vi "Actor Core.vi"(8 "error in":errorcluster, 11 "LF2R IDE in":refnum<class "LF2R IDE.lvclass">) -> (0 "error out":errorcluster, 3 "Actor out":refnum<class "Actor.lvclass">)   [LabVIEW 2018, in "LF2R IDE.lvlib" / "LF2R IDE.lvclass"]
doc: "The user interface for this panel.\n\n----\nPlease see the following web address for additional documentation and tutorial information:\nhttp://www.mooregoodideas.com/mgi-panel-manager/\n\nAuthor: Derek Trepanier\n\nCopyright (c) 2018, Moore Good Ideas, Inc.\n\nAll rights reserved.\n\nRedistribution and use in source and binary forms, with or without modification, are permitted provided that the following conditions are met:\n\n * Redistributions of source code must retain the above copyright notice, this list of conditions and the following disclaimer.\n * Redistributions in binary form must reproduce the above copyright notice, this list of conditions and the following disclaimer in the documentation and/or other materials provided with the distribution.\n * Neither the name of Moore Good Ideas, Inc. nor the names of its contributors may be used to endorse or promote products derived from this software without specific prior written permission.\n\nTHIS SOFTWARE IS PROVIDED BY THE COPYRIGHT HOLDERS AND CONTRIBUTORS \"AS IS\" AND ANY EXPRESS OR IMPLIED WARRANTIES, INCLUDING, BUT NOT LIMITED TO, THE IMPLIED WARRANTIES OF MERCHANTABILITY AND FITNESS FOR A PARTICULAR PURPOSE ARE DISCLAIMED. IN NO EVENT SHALL THE COPYRIGHT OWNER OR CONTRIBUTORS BE LIABLE FOR ANY DIRECT, INDIRECT, INCIDENTAL, SPECIAL, EXEMPLARY, OR CONSEQUENTIAL DAMAGES (INCLUDING, BUT NOT LIMITED TO, PROCUREMENT OF SUBSTITUTE GOODS OR SERVICES; LOSS OF USE, DATA, OR PROFITS; OR BUSINESS INTERRUPTION) HOWEVER CAUSED AND ON ANY THEORY OF LIABILITY, WHETHER IN CONTRACT, STRICT LIABILITY, OR TORT (INCLUDING NEGLIGENCE OR OTHERWISE) ARISING IN ANY WAY OUT OF THE USE OF THIS SOFTWARE, EVEN IF ADVISED OF THE POSSIBILITY OF SUCH DAMAGE."
uses:
  LF2R IDE.lvclass
  C:/Program Files (x86)/National Instruments/LabVIEW 2018/vi.lib/MGI/Panel Manager/Panel Actor/Panel Actor/Panel Actor.lvclass
  <vilib>/ActorFramework/Actor/Actor.lvclass
  LF2R IDE.lvclass/LF2R IDE.ctl
  <vilib>/MGI/Panel Manager/Panel Actor/Panel Actor/Panel Actor.lvclass
  D:/project/hobby/LabVIEW/LF2R/LabVIEW/Source/ScintillaNET/dll/ScintillaNET.dll
  ScintillaNET/dll/ScintillaNET.dll
panel:
  in  "File Path":path
  in  "Script":refnum<k24>(container)
  in  "Numeric":u32
  in  "Load Pic":bool
  in  "Go To":u16(ring)
  in  "Tab Control":T1(tab)
  in  "sound":string
  in  "basic_dvz":i32 caption="dvz"
  in  "basic_dvy":i32 caption="dvy"
  in  "basic_dvx":i32 caption="dvx"
  in  "basic_centery":i32 caption="centery"
  in  "basic_centerx":i32 caption="centerx"
  in  "basic_next":u32 caption="next"
  in  "basic_wait":u32 caption="wait"
  in  "basic_state":u32 caption="state"
  in  "basic_pic":u32 caption="pic"
  in  "To Next Frame":bool
  in  "basic_hit_Da":u32 caption="hit_Da"
  in  "basic_mp":i32 caption="mp"
  in  "basic_hit_Fa":u32 caption="hit_Fa"
  in  "basic_hit_Fj":u32 caption="hit_Fj"
  in  "basic_hit_Ua":u32 caption="hit_Ua"
  in  "basic_hit_Uj":u32 caption="hit_Uj"
  in  "basic_hit_Dj":u32 caption="hit_Dj"
  in  "basic_hit_ja":u32 caption="hit_ja"
  in  "basic_hit_d":u32 caption="hit_d"
  in  "basic_hit_a":u32 caption="hit_a"
  in  "basic_hit_j":u32 caption="hit_j"
  in  "bp_y":dbl caption="y"
  in  "bp_x":dbl caption="x"
  in  "w_attacking":u32 caption="attacking"
  in  "w_dvz":i32 caption="dvz"
  in  "w_dvy":i32 caption="dvy"
  in  "w_dvx":i32 caption="dvx"
  in  "w_cover":u32 caption="cover"
  in  "w_weaponact":u32 caption="weaponact"
  in  "w_y":dbl caption="y"
  in  "w_x":dbl caption="x"
  in  "w_kind":u32 caption="kind"
  in  "b_h":u32 caption="h"
  in  "b_w":u32 caption="w"
  in  "b_y":i32 caption="y"
  in  "b_x":i32 caption="x"
  in  "b_kind":u32 caption="kind"
  in  "<b> index":u32(slide) scale=0.0..10.0
  in  "i_zwidth":u32 caption="zwidth"
  in  "i_caughtact 2":u32 caption="caughtact 2"
  in  "i_catchingact 2":u32 caption="catchingact 2"
  in  "i_caughtact 1":u32 caption="caughtact 1"
  in  "i_catchingact 1":u32 caption="catchingact 1"
  in  "i_effect":u32 caption="effect"
  in  "i_injury":i32 caption="injury"
  in  "i_bdefend":i32 caption="bdefend"
  in  "i_vrest":u32 caption="vrest"
  in  "i_arest":u32 caption="arest"
  in  "i_fall":u32 caption="fall"
  in  "i_dvz":i32 caption="dvz"
  in  "i_dvy":i32 caption="dvy"
  in  "i_dvx":i32 caption="dvx"
  in  "i_h":u32 caption="h"
  in  "i_w":u32 caption="w"
  in  "i_y":i32 caption="y"
  in  "i_x":i32 caption="x"
  in  "i_kind":u32 caption="kind"
  in  "<i> index":u32(slide) scale=0.0..10.0
  in  "o_facing":i32 caption="facing"
  in  "o_oid":u32 caption="oid"
  in  "o_action":u32 caption="action"
  in  "o_kind":u32 caption="kind"
  in  "o_x":i32 caption="x"
  in  "o_y":i32 caption="y"
  in  "o_dvx":i32 caption="dvx"
  in  "o_dvy":i32 caption="dvy"
  in  "o_dvz":i32 caption="dvz"
  in  "c_cover":i32 caption="cover"
  in  "c_injury":i32 caption="injury"
  in  "c_dircontrol":i32 caption="dircontrol"
  in  "c_backhurtact":i32 caption="backhurtact"
  in  "c_fronthurtact":i32 caption="fronthurtact"
  in  "c_decrease":i32 caption="decrease"
  in  "c_hurtable":i32 caption="hurtable"
  in  "c_taction":i32 caption="taction"
  in  "c_aaction":i32 caption="aaction"
  in  "c_vaction":i32 caption="vaction"
  in  "c_y":i32 caption="y"
  in  "c_x":i32 caption="x"
  in  "c_kind":u32 caption="kind"
  in  "c_throwvx":i32 caption="throwvx"
  in  "c_throwvy":i32 caption="throwvy"
  in  "c_throwvz":i32 caption="throwvz"
  in  "c_throwinjury":i32 caption="throwinjury"
  in  "title_name":string caption="Name"
  in  "Apply Change":bool
  in  "title_num":u32 caption="Frame Num" format="%03d"
  out "Image Display":T2(plugin-control)
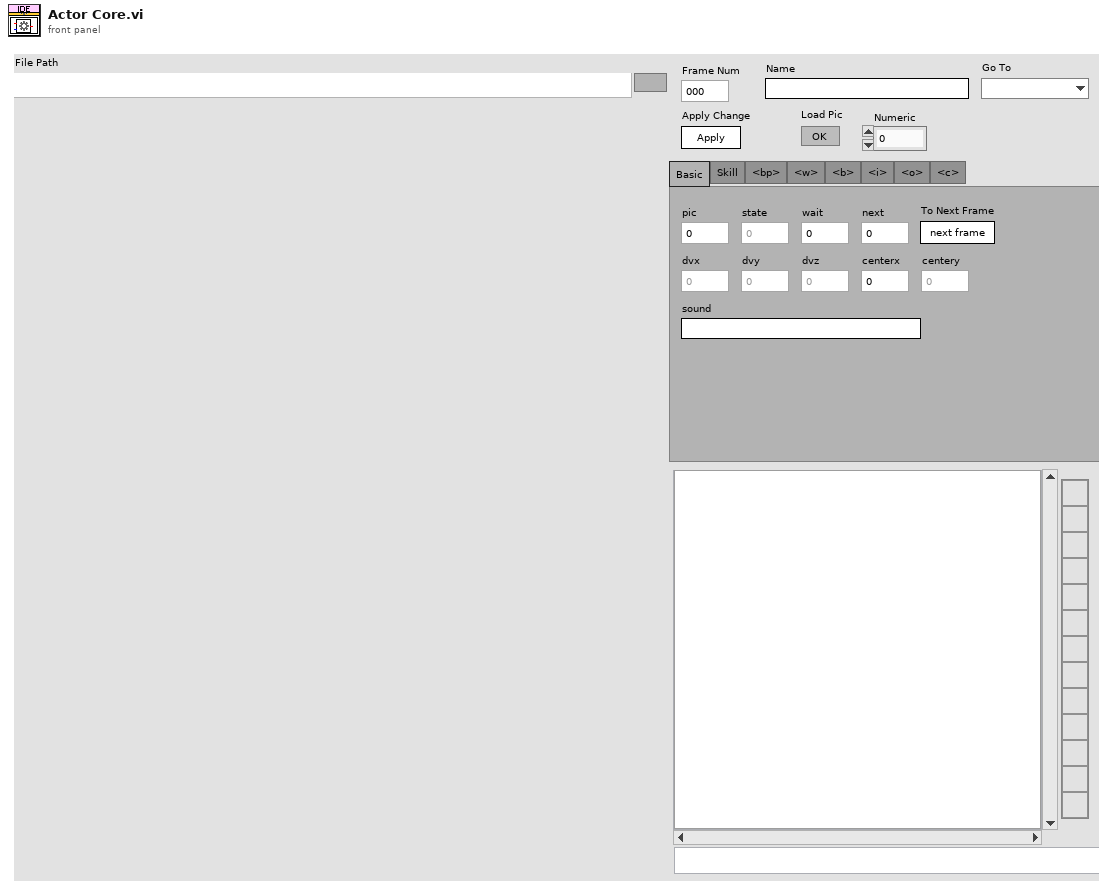
[diagram p1: front panel]
types:
  T1 = enum32{"Basic", "Skill", "<bp>", "<w>", "<b>", "<i>", "<o>", "<c>"}
  T2 = typedef "IMAQ Image.ctl" = refnum<image>
  T3 = cluster{"title_num":refnum<vi>, "title_name":refnum<vi>}
  T4 = cluster{"basic_pic":refnum<vi>, "basic_state":refnum<vi>, "basic_wait":refnum<vi>, "basic_next":refnum<vi>}
  T5 = cluster{"basic_centerx":refnum<vi>, "basic_centery":refnum<vi>}
  T6 = cluster{"basic_dvx":refnum<vi>, "basic_dvy":refnum<vi>, "basic_dvz":refnum<vi>}
  T7 = cluster{"b_kind":refnum<vi>, "b_x":refnum<vi>, "b_y":refnum<vi>, "b_w":refnum<vi>, "b_h":refnum<vi>, "<b> index":refnum<vi>}
  T8 = cluster{"w_kind":refnum<vi>, "w_x":refnum<vi>, "w_y":refnum<vi>, "w_weaponact":refnum<vi>, "w_dvx":refnum<vi>, "w_dvy":refnum<vi>, "w_dvz":refnum<vi>, "w_attacking":refnum<vi>, "w_cover":refnum<vi>}
  T9 = cluster{"basic_hit_a":refnum<vi>, "basic_hit_d":refnum<vi>, "basic_hit_j":refnum<vi>, "basic_hit_Fa":refnum<vi>, "basic_hit_Ua":refnum<vi>, "basic_hit_Da":refnum<vi>, "basic_hit_Fj":refnum<vi>, "basic_hit_Uj":refnum<vi>, "basic_hit_Dj":refnum<vi>, "basic_hit_ja":refnum<vi>}
  T10 = cluster{"o_kind":refnum<vi>, "o_x":refnum<vi>, "o_y":refnum<vi>, "o_action":refnum<vi>, "o_dvx":refnum<vi>, "o_dvy":refnum<vi>, "o_dvz":refnum<vi>, "o_oid":refnum<vi>, "o_facing":refnum<vi>}
  T11 = cluster{"i_kind":refnum<vi>, "i_x":refnum<vi>, "i_y":refnum<vi>, "i_w":refnum<vi>, "i_h":refnum<vi>, "i_dvx":refnum<vi>, "i_dvy":refnum<vi>, "i_dvz":refnum<vi>, "i_fall":refnum<vi>, "i_arest":refnum<vi>, "i_vrest":refnum<vi>, "i_bdefend":refnum<vi>, "i_injury":refnum<vi>, "i_zwidth":refnum<vi>, "i_effect":refnum<vi>, "i_catchingact 1":refnum<vi>, "i_catchingact 2":refnum<vi>, "i_caughtact 1":refnum<vi>, "i_caughtact 2":refnum<vi>, "<i> index":refnum<vi>}
  T12 = cluster{"c_kind":refnum<vi>, "c_x":refnum<vi>, "c_y":refnum<vi>, "c_injury":refnum<vi>, "c_cover":refnum<vi>, "c_vaction":refnum<vi>, "c_aaction":refnum<vi>, "c_taction":refnum<vi>, "c_hurtable":refnum<vi>, "c_decrease":refnum<vi>, "c_fronthurtact":refnum<vi>, "c_backhurtact":refnum<vi>, "c_dircontrol":refnum<vi>, "c_throwvx":refnum<vi>, "c_throwvy":refnum<vi>, "c_throwvz":refnum<vi>, "c_throwinjury":refnum<vi>}
  T13 = cluster{"Event Registration Refnum":refnum<event-registration>, "Pnl Actor":refnum<event-registration>}
  T14 = typedef "LF2R IDE.lvlib/LF2R IDE.lvclass/CMD.ctl" = enum16{"Save File"}
  T15 = cluster{"Shift":bool, "Ctrl":bool, "Alt":bool, "Cmd":bool, "Opt":bool}
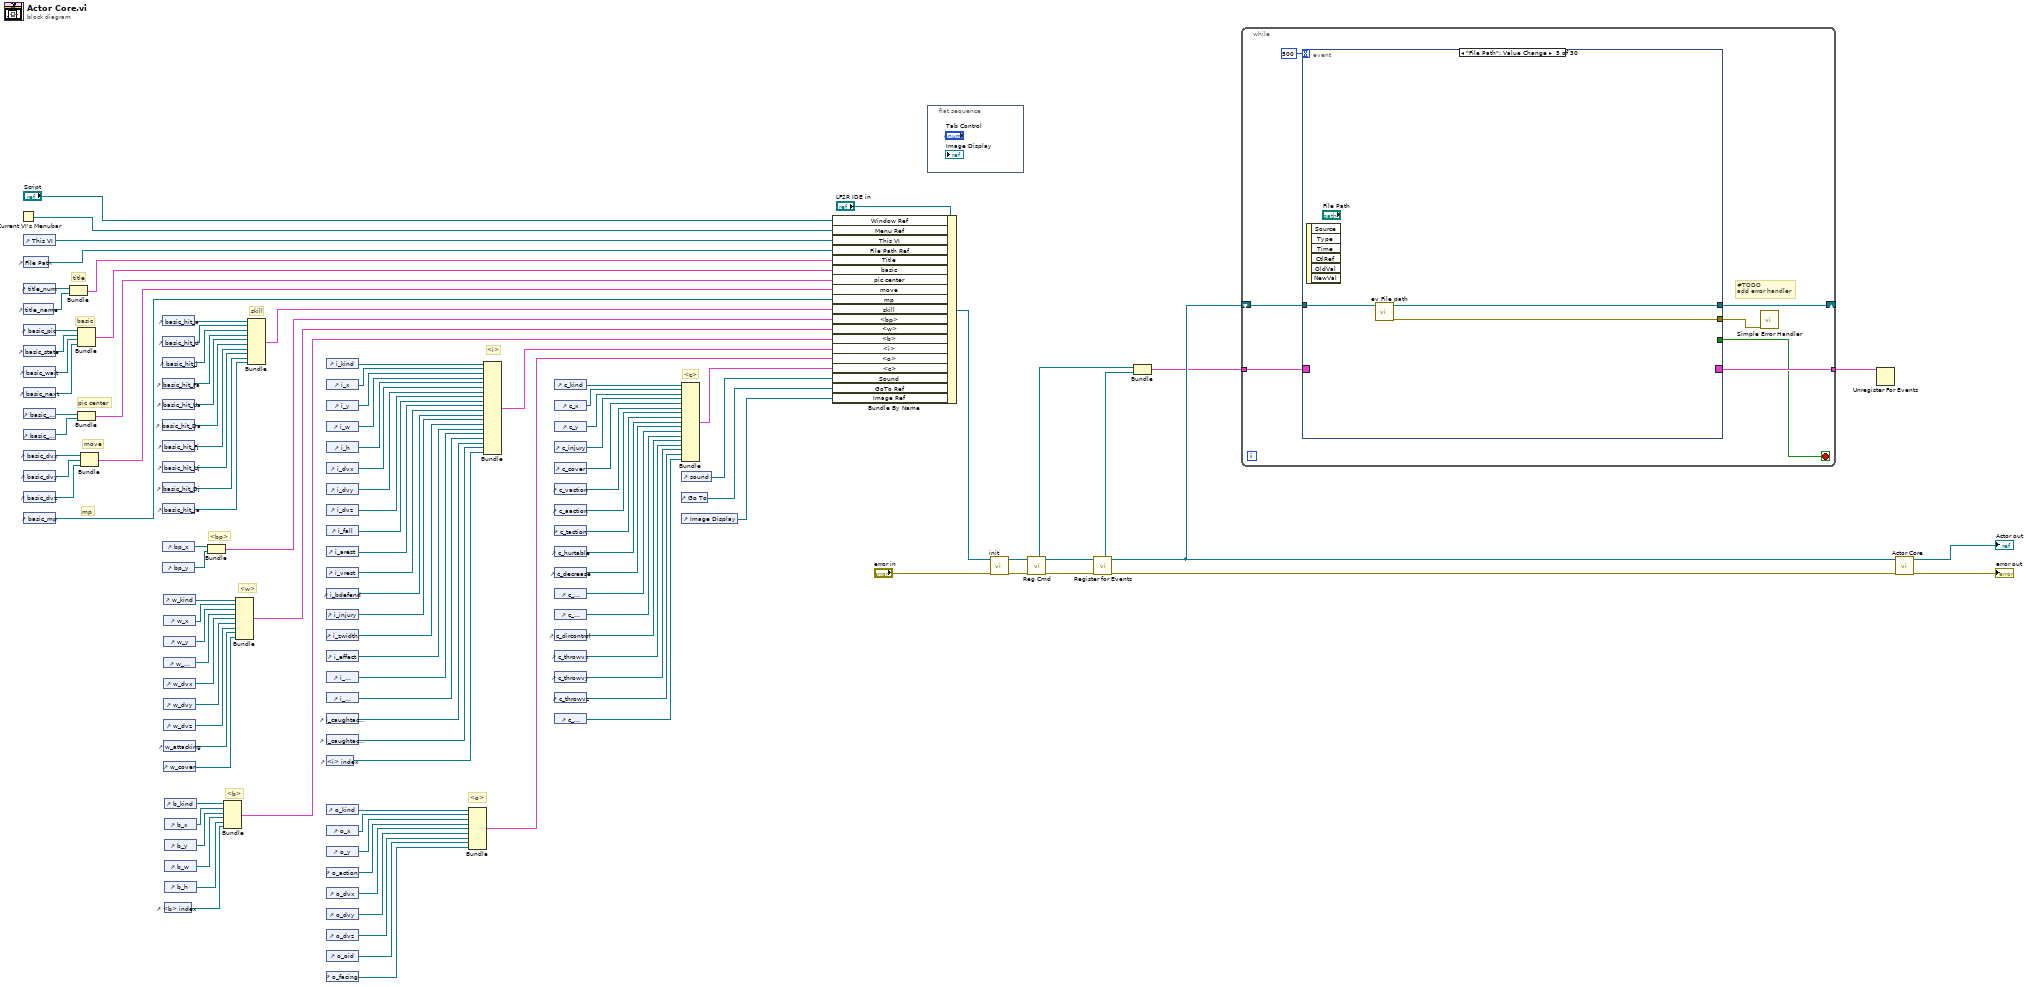
[diagram p0: block diagram]
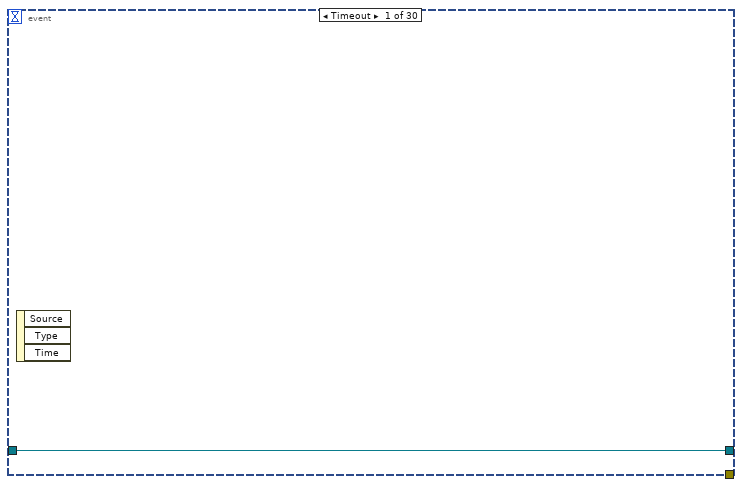
[diagram p2: hidden frame]
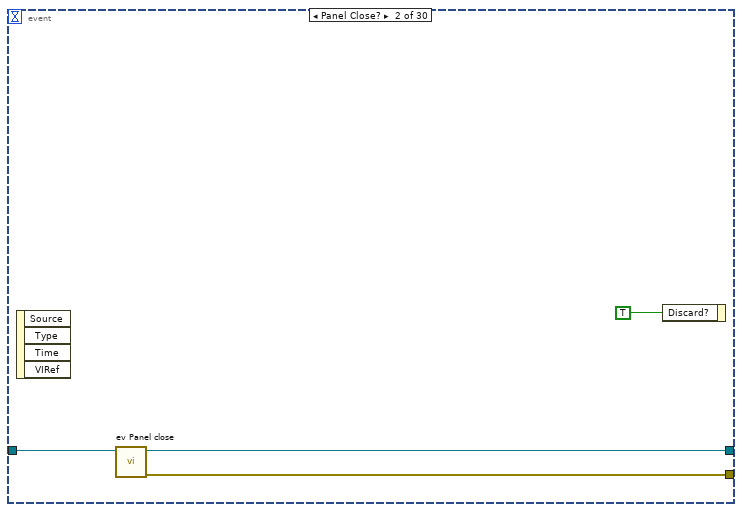
[diagram p3: hidden frame]
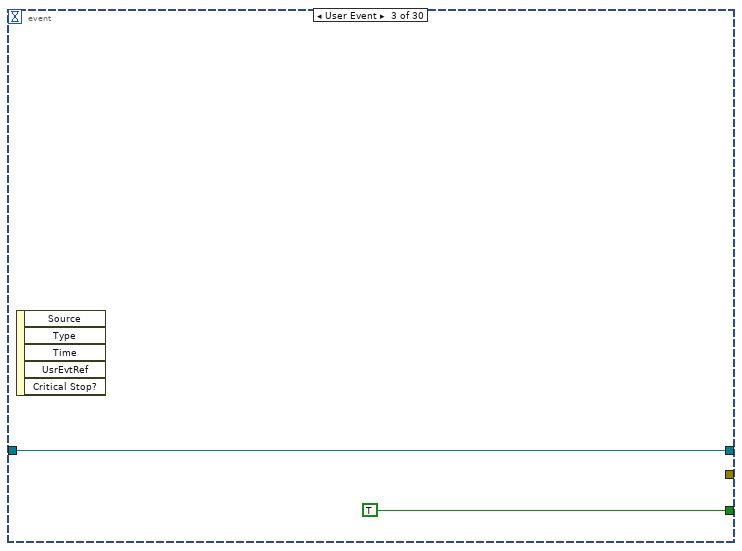
[diagram p4: hidden frame]
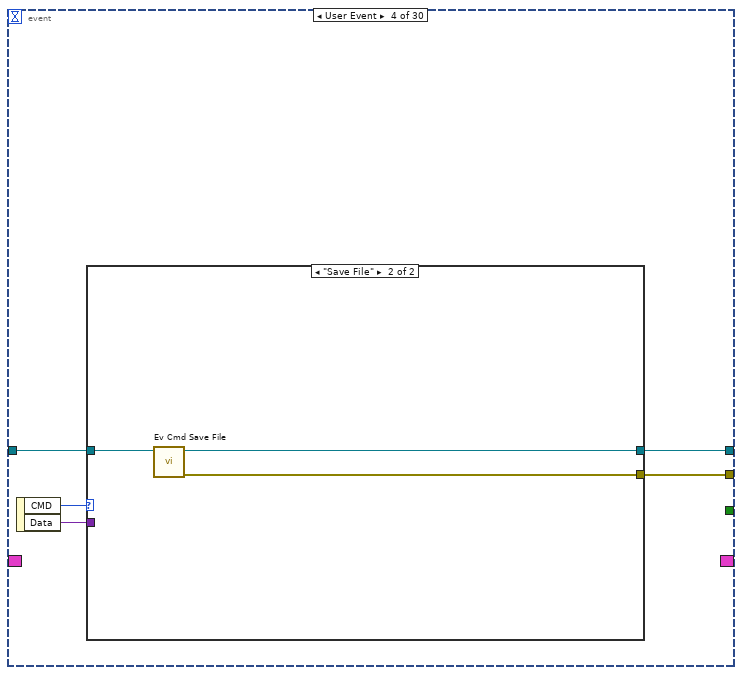
[diagram p5: hidden frame]
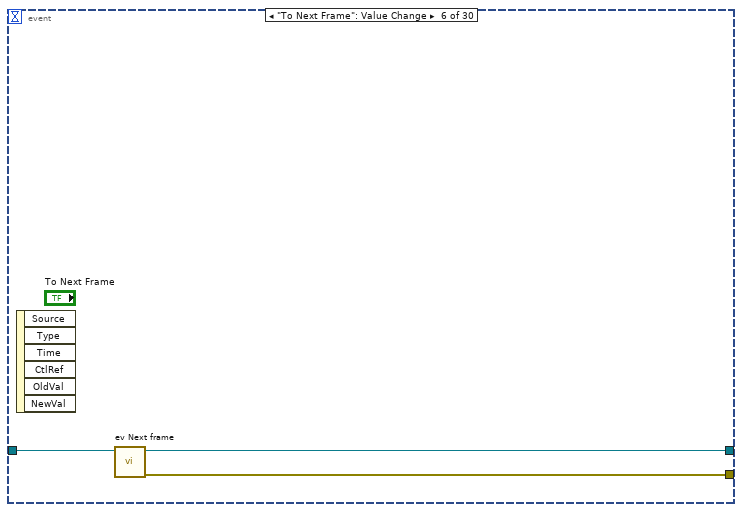
[diagram p7: hidden frame]
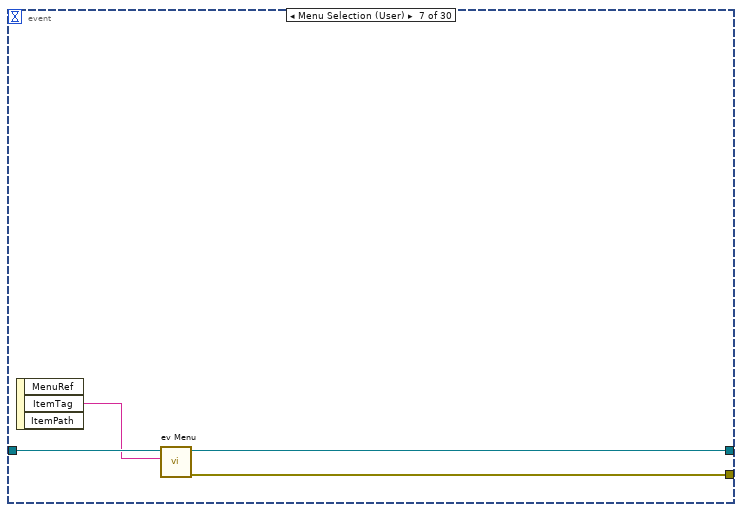
[diagram p8: hidden frame]
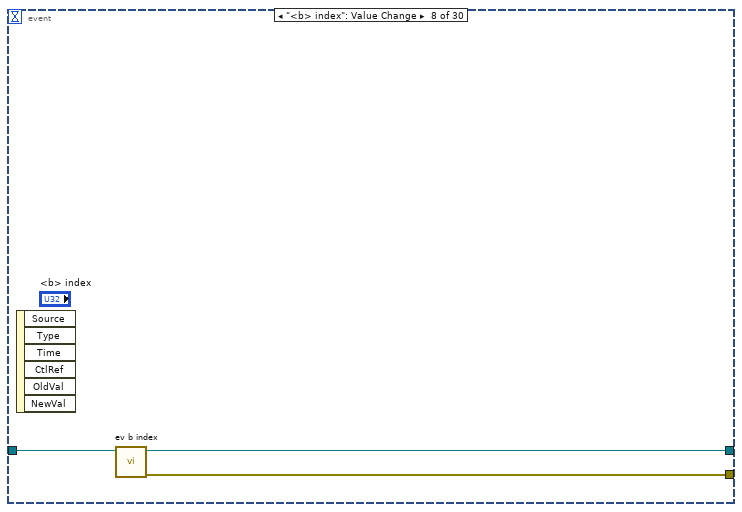
[diagram p9: hidden frame]
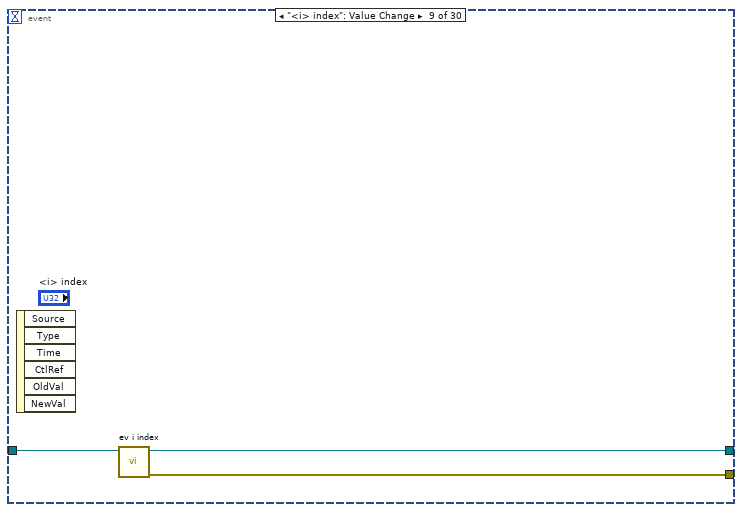
[diagram p10: hidden frame]
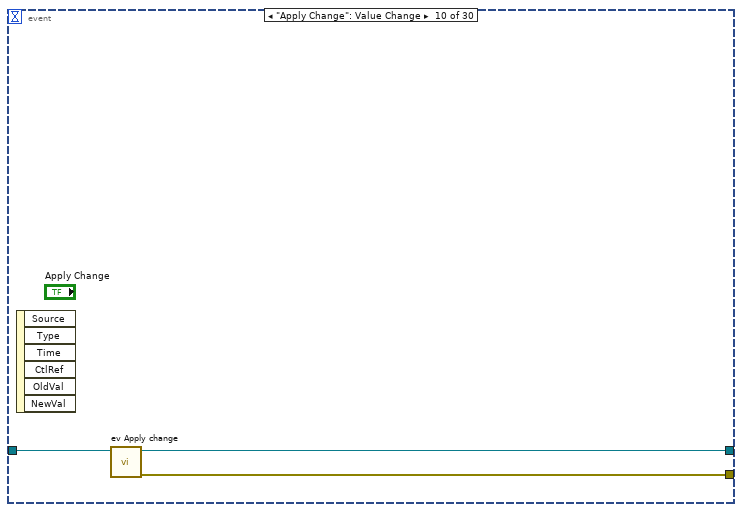
[diagram p11: hidden frame]
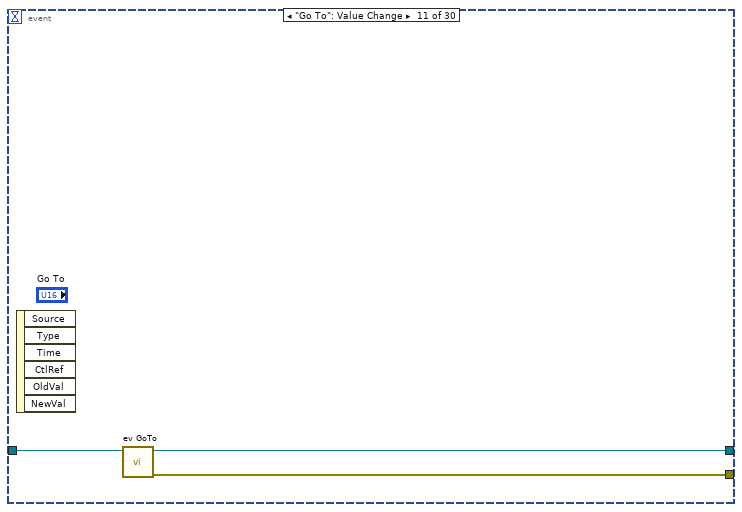
[diagram p12: hidden frame]
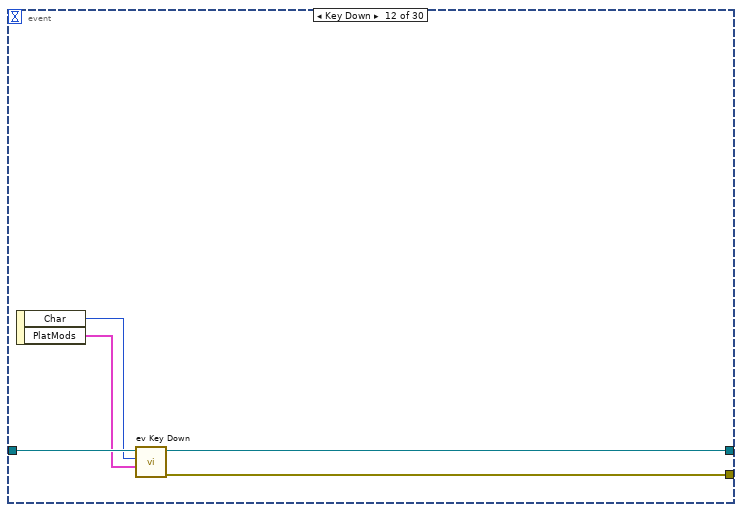
[diagram p13: hidden frame]
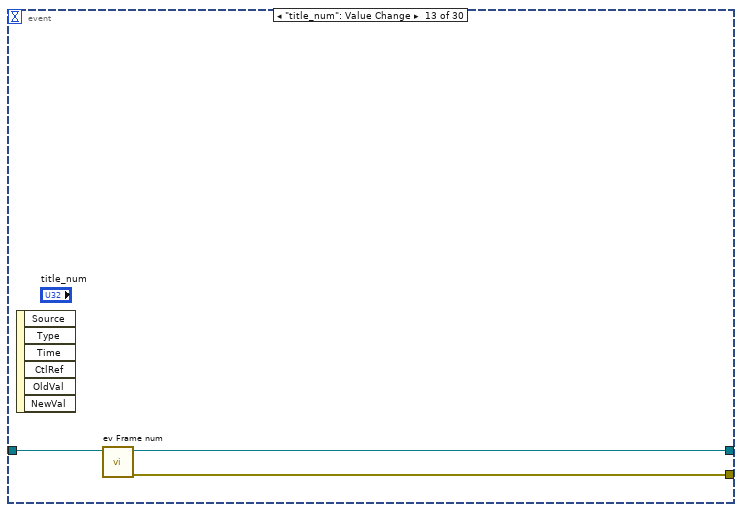
[diagram p14: hidden frame]
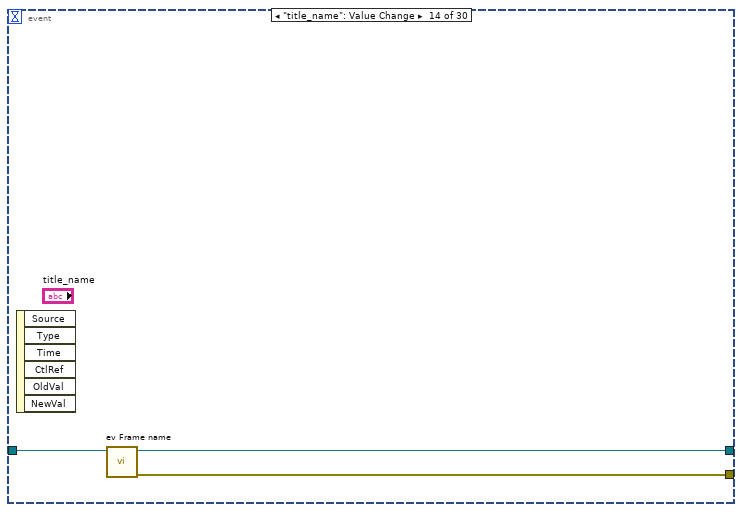
[diagram p15: hidden frame]
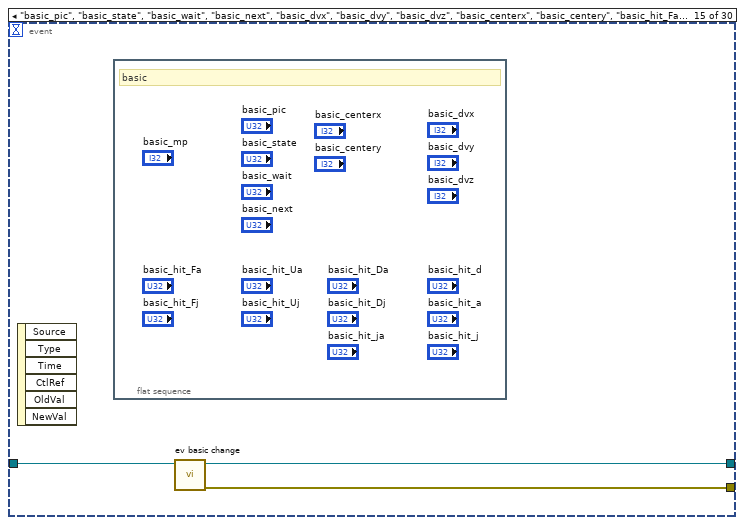
[diagram p16: hidden frame]
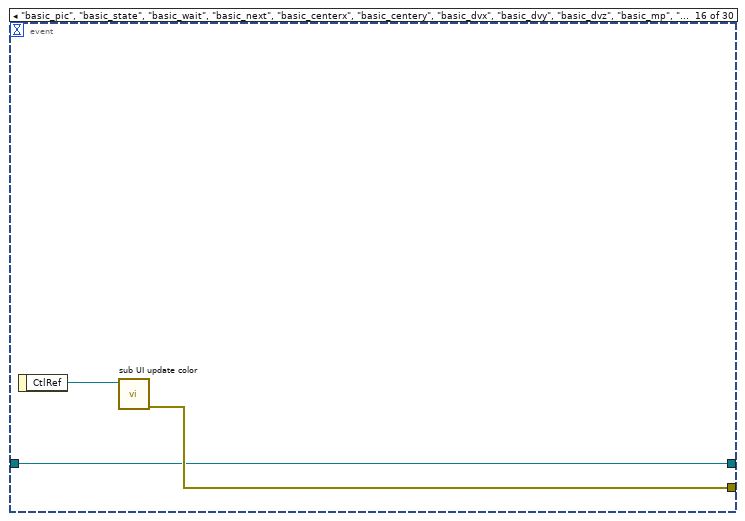
[diagram p17: hidden frame]
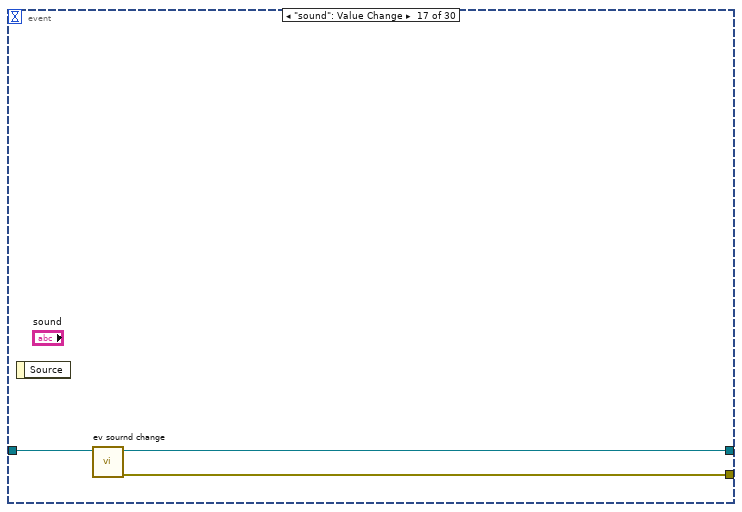
[diagram p18: hidden frame]
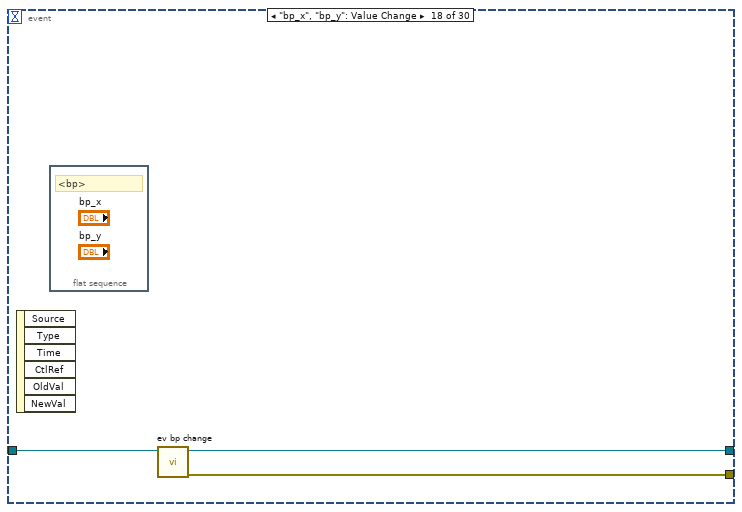
[diagram p19: hidden frame]
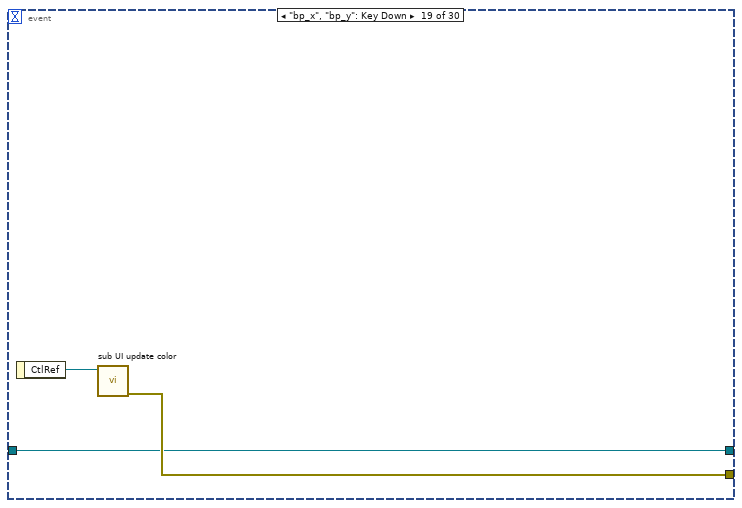
[diagram p20: hidden frame]
diagram:
  # "<c>"
  # "<o>"
  # "<i>"
  # "title"
  # "basic"
  # "pic center"
  # "move"
  # "mp"
  # "skill"
  # "<bp>"
  # "<w>"
  # "<b>"
  n1 = Current VI's Menubar() -> (w17:refnum<k9>)
  n2 = control-ref of="This VI"() -> (w18:refnum<vi>)
  n3 = control-ref of="File Path"() -> (w116:refnum<vi>)
  n4 = control-ref of="title_num"() -> (w106:refnum<vi>)
  n5 = control-ref of="title_name"() -> (w105:refnum<vi>)
  n6 = control-ref of="basic_pic"() -> (w115:refnum<vi>)
  n7 = control-ref of="basic_state"() -> (w114:refnum<vi>)
  n8 = control-ref of="basic_wait"() -> (w113:refnum<vi>)
  n9 = control-ref of="basic_next"() -> (w112:refnum<vi>)
  n10 = control-ref of="basic_centerx"() -> (w111:refnum<vi>)
  n11 = control-ref of="basic_centery"() -> (w110:refnum<vi>)
  n12 = control-ref of="basic_dvx"() -> (w109:refnum<vi>)
  n13 = control-ref of="basic_dvy"() -> (w108:refnum<vi>)
  n14 = control-ref of="basic_dvz"() -> (w107:refnum<vi>)
  n15 = control-ref of="basic_mp"() -> (w100:refnum<vi>)
  n16 = Bundle("title_num"=w106, "title_name"=w105) -> (w104:T3)  [unwired: 1 in]
  n17 = Bundle("basic_pic"=w115, "basic_state"=w114, "basic_wait"=w113, "basic_next"=w112) -> (w103:T4)  [unwired: 1 in]
  n18 = Bundle("basic_centerx"=w111, "basic_centery"=w110) -> (w102:T5)  [unwired: 1 in]
  n19 = Bundle("basic_dvx"=w109, "basic_dvy"=w108, "basic_dvz"=w107) -> (w101:T6)  [unwired: 1 in]
  n20 = control-ref of="basic_hit_a"() -> (w37:refnum<vi>)
  n21 = control-ref of="basic_hit_d"() -> (w36:refnum<vi>)
  n22 = control-ref of="basic_hit_j"() -> (w35:refnum<vi>)
  n23 = control-ref of="basic_hit_Fa"() -> (w34:refnum<vi>)
  n24 = control-ref of="basic_hit_Ua"() -> (w33:refnum<vi>)
  n25 = control-ref of="basic_hit_Da"() -> (w32:refnum<vi>)
  n26 = control-ref of="basic_hit_Fj"() -> (w31:refnum<vi>)
  n27 = control-ref of="basic_hit_Uj"() -> (w30:refnum<vi>)
  n28 = control-ref of="basic_hit_Dj"() -> (w29:refnum<vi>)
  n29 = control-ref of="basic_hit_ja"() -> (w28:refnum<vi>)
  n30 = control-ref of="bp_x"() -> (w26:refnum<vi>)
  n31 = control-ref of="bp_y"() -> (w25:refnum<vi>)
  n32 = control-ref of="w_kind"() -> (w99:refnum<vi>)
  n33 = control-ref of="w_x"() -> (w98:refnum<vi>)
  n34 = control-ref of="w_y"() -> (w97:refnum<vi>)
  n35 = control-ref of="w_weaponact"() -> (w96:refnum<vi>)
  n36 = control-ref of="w_dvx"() -> (w95:refnum<vi>)
  n37 = control-ref of="w_dvy"() -> (w94:refnum<vi>)
  n38 = control-ref of="w_dvz"() -> (w93:refnum<vi>)
  n39 = control-ref of="w_attacking"() -> (w92:refnum<vi>)
  n40 = control-ref of="w_cover"() -> (w24:refnum<vi>)
  n41 = control-ref of="b_kind"() -> (w91:refnum<vi>)
  n42 = control-ref of="b_x"() -> (w90:refnum<vi>)
  n43 = control-ref of="b_y"() -> (w89:refnum<vi>)
  n44 = control-ref of="b_w"() -> (w88:refnum<vi>)
  n45 = control-ref of="b_h"() -> (w87:refnum<vi>)
  n46 = control-ref of="<b> index"() -> (w40:refnum<vi>)
  n47 = Bundle("bp_x"=w26, "bp_y"=w25) -> (w61:cluster{"bp_x":refnum<vi>, "bp_y":refnum<vi>})  [unwired: 1 in]
  n48 = Bundle("b_kind"=w91, "b_x"=w90, "b_y"=w89, "b_w"=w88, "b_h"=w87, "<b> index"=w40) -> (w59:T7)  [unwired: 1 in]
  n49 = Bundle("w_kind"=w99, "w_x"=w98, "w_y"=w97, "w_weaponact"=w96, "w_dvx"=w95, "w_dvy"=w94, "w_dvz"=w93, "w_attacking"=w92, "w_cover"=w24) -> (w60:T8)  [unwired: 1 in]
  n50 = Bundle("basic_hit_a"=w37, "basic_hit_d"=w36, "basic_hit_j"=w35, "basic_hit_Fa"=w34, "basic_hit_Ua"=w33, "basic_hit_Da"=w32, "basic_hit_Fj"=w31, "basic_hit_Uj"=w30, "basic_hit_Dj"=w29, "basic_hit_ja"=w28) -> (w27:T9)  [unwired: 1 in]
  n51 = control-ref of="i_kind"() -> (w86:refnum<vi>)
  n52 = control-ref of="i_x"() -> (w85:refnum<vi>)
  n53 = control-ref of="i_y"() -> (w84:refnum<vi>)
  n54 = control-ref of="i_w"() -> (w83:refnum<vi>)
  n55 = control-ref of="i_h"() -> (w82:refnum<vi>)
  n56 = control-ref of="i_dvx"() -> (w81:refnum<vi>)
  n57 = control-ref of="i_dvy"() -> (w80:refnum<vi>)
  n58 = control-ref of="i_dvz"() -> (w79:refnum<vi>)
  n59 = control-ref of="i_fall"() -> (w78:refnum<vi>)
  n60 = control-ref of="i_arest"() -> (w77:refnum<vi>)
  n61 = control-ref of="i_vrest"() -> (w76:refnum<vi>)
  n62 = control-ref of="i_bdefend"() -> (w75:refnum<vi>)
  n63 = control-ref of="i_injury"() -> (w74:refnum<vi>)
  n64 = control-ref of="i_zwidth"() -> (w23:refnum<vi>)
  n65 = control-ref of="i_effect"() -> (w73:refnum<vi>)
  n66 = control-ref of="i_catchingact 1"() -> (w72:refnum<vi>)
  n67 = control-ref of="i_catchingact 2"() -> (w42:refnum<vi>)
  n68 = control-ref of="i_caughtact 1"() -> (w71:refnum<vi>)
  n69 = control-ref of="i_caughtact 2"() -> (w41:refnum<vi>)
  n70 = control-ref of="<i> index"() -> (w38:refnum<vi>)
  n71 = control-ref of="o_kind"() -> (w70:refnum<vi>)
  n72 = control-ref of="o_x"() -> (w69:refnum<vi>)
  n73 = control-ref of="o_y"() -> (w68:refnum<vi>)
  n74 = control-ref of="o_action"() -> (w67:refnum<vi>)
  n75 = control-ref of="o_dvx"() -> (w66:refnum<vi>)
  n76 = control-ref of="o_dvy"() -> (w65:refnum<vi>)
  n77 = control-ref of="o_dvz"() -> (w64:refnum<vi>)
  n78 = control-ref of="o_oid"() -> (w63:refnum<vi>)
  n79 = control-ref of="o_facing"() -> (w62:refnum<vi>)
  n80 = Bundle("o_kind"=w70, "o_x"=w69, "o_y"=w68, "o_action"=w67, "o_dvx"=w66, "o_dvy"=w65, "o_dvz"=w64, "o_oid"=w63, "o_facing"=w62) -> (w58:T10)  [unwired: 1 in]
  n81 = Bundle("i_kind"=w86, "i_x"=w85, "i_y"=w84, "i_w"=w83, "i_h"=w82, "i_dvx"=w81, "i_dvy"=w80, "i_dvz"=w79, "i_fall"=w78, "i_arest"=w77, "i_vrest"=w76, "i_bdefend"=w75, "i_injury"=w74, "i_zwidth"=w23, "i_effect"=w73, "i_catchingact 1"=w72, "i_catchingact 2"=w42, "i_caughtact 1"=w71, "i_caughtact 2"=w41, "<i> index"=w38) -> (w39:T11)  [unwired: 1 in]
  n82 = control-ref of="c_kind"() -> (w57:refnum<vi>)
  n83 = control-ref of="c_x"() -> (w56:refnum<vi>)
  n84 = control-ref of="c_y"() -> (w55:refnum<vi>)
  n85 = control-ref of="c_injury"() -> (w22:refnum<vi>)
  n86 = control-ref of="c_cover"() -> (w21:refnum<vi>)
  n87 = control-ref of="c_vaction"() -> (w54:refnum<vi>)
  n88 = control-ref of="c_aaction"() -> (w53:refnum<vi>)
  n89 = control-ref of="c_taction"() -> (w52:refnum<vi>)
  n90 = control-ref of="c_hurtable"() -> (w51:refnum<vi>)
  n91 = control-ref of="c_decrease"() -> (w50:refnum<vi>)
  n92 = control-ref of="c_fronthurtact"() -> (w49:refnum<vi>)
  n93 = control-ref of="c_backhurtact"() -> (w48:refnum<vi>)
  n94 = control-ref of="c_dircontrol"() -> (w47:refnum<vi>)
  n95 = control-ref of="c_throwvx"() -> (w46:refnum<vi>)
  n96 = control-ref of="c_throwvy"() -> (w45:refnum<vi>)
  n97 = control-ref of="c_throwvz"() -> (w44:refnum<vi>)
  n98 = control-ref of="c_throwinjury"() -> (w43:refnum<vi>)
  n99 = Bundle("c_kind"=w57, "c_x"=w56, "c_y"=w55, "c_injury"=w22, "c_cover"=w21, "c_vaction"=w54, "c_aaction"=w53, "c_taction"=w52, "c_hurtable"=w51, "c_decrease"=w50, "c_fronthurtact"=w49, "c_backhurtact"=w48, "c_dircontrol"=w47, "c_throwvx"=w46, "c_throwvy"=w45, "c_throwvz"=w44, "c_throwinjury"=w43) -> (w20:T12)  [unwired: 1 in]
  n100 = control-ref of="sound"() -> (w19:refnum<vi>)
  n101 = control-ref of="Go To"() -> (w2:refnum<vi>)
  n102 = control-ref of="Image Display"() -> (w1:refnum<vi>)
  n103 = Bundle By Name(cluster="LF2R IDE in", "Window Ref"="Script", "Menu Ref"=w17, "This VI"=w18, "File Path Ref"=w116, "Title"=w104, "basic"=w103, "pic center"=w102, "move"=w101, "mp"=w100, "skill"=w27, "<bp>"=w61, "<w>"=w60, "<b>"=w59, "<i>"=w39, "<o>"=w58, "<c>"=w20, "Sound"=w19, "GoTo Ref"=w2, "Image Ref"=w1) -> (w12:refnum<class "LF2R IDE.lvclass">)
  n104 = flat-sequence {
    frame #0 {
    }
  }
  n105 = call "init.vi"("error in (no error)"="error in", "IDE simple in"=w12) -> ("error out"=w8:errorcluster, "IDE simple out"=w9:refnum<class "LF2R IDE.lvclass">)  [unwired: 8 in]
  n106 = call "Reg Cmd.vi"("error in (no error)"=w8, "LF2R IDE in"=w9) -> ("error out"=w6:errorcluster, "LF2R IDE out"=w7:refnum<class "LF2R IDE.lvclass">, "Event Registration Refnum"=w5:refnum<event-registration>)  [unwired: 7 in]
  n107 = call <vilib>:"Register for Events.vi"("Error In"=w6, "Panel Actor in"=w7) -> ("Error Out"=w15:errorcluster, "Panel Actor out"=w14:refnum<class "LF2R IDE.lvclass">, "Pnl Actor"=w4:refnum<event-registration>)  [unwired: 6 in, 1 out]
  n108 = Bundle("Event Registration Refnum"=w5, "Pnl Actor"=w4) -> (w3:T13)  [unwired: 1 in]
  n109 = while {
    shift-right: [w124] -> _
    shift-left: w14 -> [w125]
    tunnel: [w123] -> w13
    tunnel: w3 -> [w120]
    stop <- w119 stop-if-true
    # "#TODO\nadd error handler"
    n110 = event shown="[4] \"File Path\": Value Change" {
      selector: w120 -> [_ _ _ _ _ _ _ _ _ _ _ _ _ _ _ _ _ _ _ _ _ _ _ _ _ _ _ _ _ _]
      dyn-events: [_ _ _ _ _ _ _ _ _ _ _ _ _ _ _ _ _ _ _ _ _ _ _ _ _ _ _ _ _ _] -> w123
      timeout: 500 -> [_ _ _ _ _ _ _ _ _ _ _ _ _ _ _ _ _ _ _ _ _ _ _ _ _ _ _ _ _ _]
      tunnel: w125 -> [w126 w129 w132 w136 w144 w147 w151 w154 w157 w160 w163 w168 w171 w174 w177 w178 w183 w186 w187 w192 w194 w198 w199 w204 w206 w210 w211 w216 w218 w223]
      tunnel: [w126 w127 w132 w135 w142 w146 w150 w153 w156 w159 w161 w166 w169 w173 w176 w178 w181 w185 w187 w191 w194 w196 w199 w202 w206 w209 w211 w214 w218 w221] -> w124
      tunnel: [_ _ TRUE ("Stop") _ _ _ _ _ _ _ _ _ _ _ _ _ _ _ _ _ _ _ _ _ _ _ _ _ _ _] -> w119
      tunnel: [_ w128 _ w133 w143 w145 w149 w152 w155 w158 w162 w167 w170 w172 w175 w179 w182 w184 w188 w190 w193 w197 w200 w203 w205 w208 w212 w215 w217 w222] -> w122
      event Timeout {
        n111 = event-data() -> ()  [unwired: 1 in, 3 out]
      }
      event Panel Close? {
        n112 = event-data() -> ()  [unwired: 1 in, 4 out]
        n113 = call "ev Panel close.vi"("LF2R IDE in"=w129) -> ("error out"=w128:errorcluster, "LF2R IDE out"=w127:refnum<class "LF2R IDE.lvclass">)  [unwired: 9 in]
        n114 = event-data("Discard?"=TRUE) -> ()  [unwired: 1 in, 1 out]
      }
      event User Event {
        n115 = event-data() -> ()  [unwired: 1 in, 5 out]
      }
      event User Event {
        n116 = event-data() -> ("CMD"=w137:T14, "Data"=w134:variant)  [unwired: 1 in]
        n117 = case shown="\"Save File\"" w137 {
          tunnel: w136 -> [w138 w141]
          tunnel: [w138 w140] -> w135
          tunnel: w134 -> [_ _]
          tunnel: [_ w139] -> w133
          frame Default {
          }
          frame "Save File" {
            n118 = call "Ev Cmd Save File.vi"("LF2R IDE in"=w141) -> ("error out"=w139:errorcluster, "LF2R IDE out"=w140:refnum<class "LF2R IDE.lvclass">)  [unwired: 9 in]
          }
        }
      }
      event "File Path": Value Change {
        n119 = event-data() -> ()  [unwired: 1 in, 6 out]
        n120 = call "ev File path.vi"("LF2R IDE in"=w144) -> ("error out"=w143:errorcluster, "LF2R IDE out"=w142:refnum<class "LF2R IDE.lvclass">)  [unwired: 9 in]
      }
      event "To Next Frame": Value Change {
        n121 = event-data() -> ()  [unwired: 1 in, 6 out]
        n122 = call "ev Next frame.vi"("IDE simple in"=w147) -> ("error out"=w145:errorcluster, "IDE simple out"=w146:refnum<class "LF2R IDE.lvclass">)  [unwired: 9 in]
      }
      event Menu Selection (User) {
        n123 = event-data() -> ("ItemTag"=w148:string)  [unwired: 1 in, 2 out]
        n124 = call "ev Menu.vi"("ItemTag"=w148, "LF2R IDE in"=w151) -> ("error out"=w149:errorcluster, "LF2R IDE out"=w150:refnum<class "LF2R IDE.lvclass">)  [unwired: 8 in]
      }
      event "<b> index": Value Change {
        n125 = event-data() -> ()  [unwired: 1 in, 6 out]
        n126 = call "ev b index.vi"("IDE simple in"=w154) -> ("error out"=w152:errorcluster, "IDE simple out"=w153:refnum<class "LF2R IDE.lvclass">)  [unwired: 9 in]
      }
      event "<i> index": Value Change {
        n127 = event-data() -> ()  [unwired: 1 in, 6 out]
        n128 = call "ev i index.vi"("IDE simple in"=w157) -> ("error out"=w155:errorcluster, "IDE simple out"=w156:refnum<class "LF2R IDE.lvclass">)  [unwired: 9 in]
      }
      event "Apply Change": Value Change {
        n129 = event-data() -> ()  [unwired: 1 in, 6 out]
        n130 = call "ev Apply change.vi"("IDE simple in"=w160) -> ("error out"=w158:errorcluster, "IDE simple out"=w159:refnum<class "LF2R IDE.lvclass">)  [unwired: 9 in]
      }
      event "Go To": Value Change {
        n131 = event-data() -> ()  [unwired: 1 in, 6 out]
        n132 = call "ev GoTo.vi"("LF2R IDE in"=w163) -> ("error out"=w162:errorcluster, "LF2R IDE out"=w161:refnum<class "LF2R IDE.lvclass">)  [unwired: 9 in]
      }
      event Key Down {
        n133 = event-data() -> ("Char"=w165:i16, "PlatMods"=w164:T15)  [unwired: 1 in]
        n134 = call "ev Key Down.vi"("PlatMods"=w164, "Char"=w165, "LF2R IDE in"=w168) -> ("error out"=w167:errorcluster, "LF2R IDE out"=w166:refnum<class "LF2R IDE.lvclass">)  [unwired: 7 in]
      }
      event "title_num": Value Change {
        n135 = event-data() -> ()  [unwired: 1 in, 6 out]
        n136 = call "ev Frame num.vi"("IDE simple in"=w171) -> ("error out"=w170:errorcluster, "IDE simple out"=w169:refnum<class "LF2R IDE.lvclass">)  [unwired: 9 in]
      }
      event "title_name": Value Change {
        n137 = event-data() -> ()  [unwired: 1 in, 6 out]
        n138 = call "ev Frame name.vi"("LF2R IDE in"=w174) -> ("error out"=w172:errorcluster, "LF2R IDE out"=w173:refnum<class "LF2R IDE.lvclass">)  [unwired: 9 in]
      }
      event "basic_pic", "basic_state", "basic_wait", "basic_next", "basic_dvx", "basic_dvy", "basic_dvz", "basic_centerx", "basic_centery", "basic_hit_Fa", "basic_hit_Fj", "basic_hit_Ua", "basic_hit_Uj", "basic_hit_Dj", "basic_hit_ja", "basic_hit_d", "basic_hit_a", "basic_hit_j", "basic_hit_Da", "basic_mp": Value Change {
        n139 = event-data() -> ()  [unwired: 1 in, 6 out]
        n140 = flat-sequence {
          frame #0 {
            # "basic"
          }
        }
        n141 = call "ev basic change.vi"("IDE simple in"=w177) -> ("error out"=w175:errorcluster, "IDE simple out"=w176:refnum<class "LF2R IDE.lvclass">)  [unwired: 9 in]
      }
      event "basic_pic", "basic_state", "basic_wait", "basic_next", "basic_centerx", "basic_centery", "basic_dvx", "basic_dvy", "basic_dvz", "basic_mp", "basic_hit_Fa", "basic_hit_Fj", "basic_hit_Ua", "basic_hit_Uj", "basic_hit_Dj", "basic_hit_ja", "basic_hit_d", "basic_hit_a", "basic_hit_j", "basic_hit_Da": Key Down {
        n142 = event-data() -> ("CtlRef"=w180:refnum<vi>)  [unwired: 1 in]
        n143 = call "sub UI update color.vi"("Num ref"=w180) -> ("error out"=w179:errorcluster)  [unwired: 10 in]
      }
      event "sound": Value Change {
        n144 = event-data() -> ()  [unwired: 1 in, 1 out]
        n145 = call "ev sournd change.vi"("IDE simple in"=w183) -> ("error out"=w182:errorcluster, "IDE simple out"=w181:refnum<class "LF2R IDE.lvclass">)  [unwired: 9 in]
      }
      event "bp_x", "bp_y": Value Change {
        n146 = event-data() -> ()  [unwired: 1 in, 6 out]
        n147 = flat-sequence {
          frame #0 {
            # "<bp>"
          }
        }
        n148 = call "ev bp change.vi"("IDE simple in"=w186) -> ("error out"=w184:errorcluster, "IDE simple out"=w185:refnum<class "LF2R IDE.lvclass">)  [unwired: 9 in]
      }
      event "bp_x", "bp_y": Key Down {
        n149 = event-data() -> ("CtlRef"=w189:refnum<vi>)  [unwired: 1 in]
        n150 = call "sub UI update color.vi"("Num ref"=w189) -> ("error out"=w188:errorcluster)  [unwired: 10 in]
      }
      event "w_kind", "w_x", "w_y", "w_weaponact", "w_cover", "w_dvx", "w_dvy", "w_dvz", "w_attacking": Value Change {
        n151 = event-data() -> ()  [unwired: 1 in, 6 out]
        n152 = flat-sequence {
          frame #0 {
            # "<w>"
          }
        }
        n153 = call "ev w change.vi"("IDE simple in"=w192) -> ("error out"=w190:errorcluster, "IDE simple out"=w191:refnum<class "LF2R IDE.lvclass">)  [unwired: 9 in]
      }
      event "w_kind", "w_x", "w_y", "w_weaponact", "w_cover", "w_dvx", "w_dvy", "w_dvz", "w_attacking": Key Down {
        n154 = event-data() -> ("CtlRef"=w195:refnum<vi>)  [unwired: 1 in]
        n155 = call "sub UI update color.vi"("Num ref"=w195) -> ("error out"=w193:errorcluster)  [unwired: 10 in]
      }
      event "b_kind", "b_x", "b_y", "b_w", "b_h": Value Change {
        n156 = event-data() -> ()  [unwired: 1 in, 6 out]
        n157 = flat-sequence {
          frame #0 {
            # "<b>"
          }
        }
        n158 = call "ev b change.vi"("IDE simple in"=w198) -> ("error out"=w197:errorcluster, "IDE simple out"=w196:refnum<class "LF2R IDE.lvclass">)  [unwired: 9 in]
      }
      event "b_kind", "b_x", "b_y", "b_w", "b_h": Key Down {
        n159 = event-data() -> ("CtlRef"=w201:refnum<vi>)  [unwired: 1 in]
        n160 = call "sub UI update color.vi"("Num ref"=w201) -> ("error out"=w200:errorcluster)  [unwired: 10 in]
      }
      event "i_kind", "i_x", "i_y", "i_w", "i_h", "i_dvx", "i_dvy", "i_dvz", "i_fall", "i_arest", "i_vrest", "i_bdefend", "i_injury", "i_effect", "i_catchingact 1", "i_caughtact 1", "i_catchingact 2", "i_caughtact 2", "i_zwidth": Value Change {
        n161 = event-data() -> ()  [unwired: 1 in, 6 out]
        n162 = flat-sequence {
          frame #0 {
            # "<i>"
          }
        }
        n163 = call "ev i change.vi"("IDE simple in"=w204) -> ("error out"=w203:errorcluster, "IDE simple out"=w202:refnum<class "LF2R IDE.lvclass">)  [unwired: 9 in]
      }
      event "i_kind", "i_x", "i_y", "i_w", "i_h", "i_dvx", "i_dvy", "i_dvz", "i_fall", "i_arest", "i_vrest", "i_bdefend", "i_injury", "i_effect", "i_catchingact 1", "i_caughtact 1", "i_catchingact 2", "i_caughtact 2", "i_zwidth": Key Down {
        n164 = event-data() -> ("CtlRef"=w207:refnum<vi>)  [unwired: 1 in]
        n165 = call "sub UI update color.vi"("Num ref"=w207) -> ("error out"=w205:errorcluster)  [unwired: 10 in]
      }
      event "o_kind", "o_x", "o_y", "o_dvx", "o_dvy", "o_dvz", "o_action", "o_oid", "o_facing": Value Change {
        n166 = event-data() -> ()  [unwired: 1 in, 1 out]
        n167 = flat-sequence {
          frame #0 {
            # "<o>"
          }
        }
        n168 = call "ev o change.vi"("IDE simple in"=w210) -> ("error out"=w208:errorcluster, "IDE simple out"=w209:refnum<class "LF2R IDE.lvclass">)  [unwired: 9 in]
      }
      event "o_kind", "o_x", "o_y", "o_dvx", "o_dvy", "o_dvz", "o_action", "o_oid", "o_facing": Key Down {
        n169 = event-data() -> ("CtlRef"=w213:refnum<vi>)  [unwired: 1 in]
        n170 = call "sub UI update color.vi"("Num ref"=w213) -> ("error out"=w212:errorcluster)  [unwired: 10 in]
      }
      event "c_kind", "c_x", "c_y", "c_vaction", "c_aaction", "c_taction", "c_hurtable", "c_decrease", "c_fronthurtact", "c_backhurtact", "c_dircontrol", "c_throwvx", "c_throwvy", "c_throwvz", "c_throwinjury", "c_injury", "c_cover": Value Change {
        n171 = event-data() -> ()  [unwired: 1 in, 1 out]
        n172 = flat-sequence {
          frame #0 {
            # "<c>"
          }
        }
        n173 = call "ev c change.vi"("IDE simple in"=w216) -> ("error out"=w215:errorcluster, "IDE simple out"=w214:refnum<class "LF2R IDE.lvclass">)  [unwired: 9 in]
      }
      event "c_kind", "c_x", "c_y", "c_vaction", "c_aaction", "c_taction", "c_hurtable", "c_decrease", "c_fronthurtact", "c_backhurtact", "c_dircontrol", "c_throwvx", "c_throwvy", "c_throwvz", "c_throwinjury", "c_injury", "c_cover": Key Down {
        n174 = event-data() -> ("CtlRef"=w219:refnum<vi>)  [unwired: 1 in]
        n175 = call "sub UI update color.vi"("Num ref"=w219) -> ("error out"=w217:errorcluster)  [unwired: 10 in]
      }
      event "Load Pic": Value Change {
        n176 = event-data() -> ()  [unwired: 1 in, 1 out]
        n177 = call "Act Load Pic.vi"("pic num"="Numeric", "LF2R IDE in"=w223) -> ("error out"=w222:errorcluster, "LF2R IDE out"=w221:refnum<class "LF2R IDE.lvclass">)  [unwired: 8 in]
      }
    }
    n178 = call <vilib>:"Simple Error Handler.vi"("error in (no error)"=w122) -> ()  [unwired: 4 in, 5 out]
  }
  n179 = Unregister For Events(event registration refnum=w13) -> ()  [unwired: 1 in, 1 out]
  n180 = call-parent "Actor Core.vi"("error in"=w15, "Panel Actor in"=w14) -> ("error out"=→"error out":errorcluster, "Actor out"=→"Actor out":refnum<class "Actor.lvclass">)  [unwired: 8 in]
